vi "histo_alerte.vi"(8 "Error in (no error)":errorcluster, 11 "Connection In":refnum<k7>) -> (0 "Error out":errorcluster, 2 "Table":string[][](table), 3 "Connection Out":refnum<k7>)   [LabVIEW 2019]
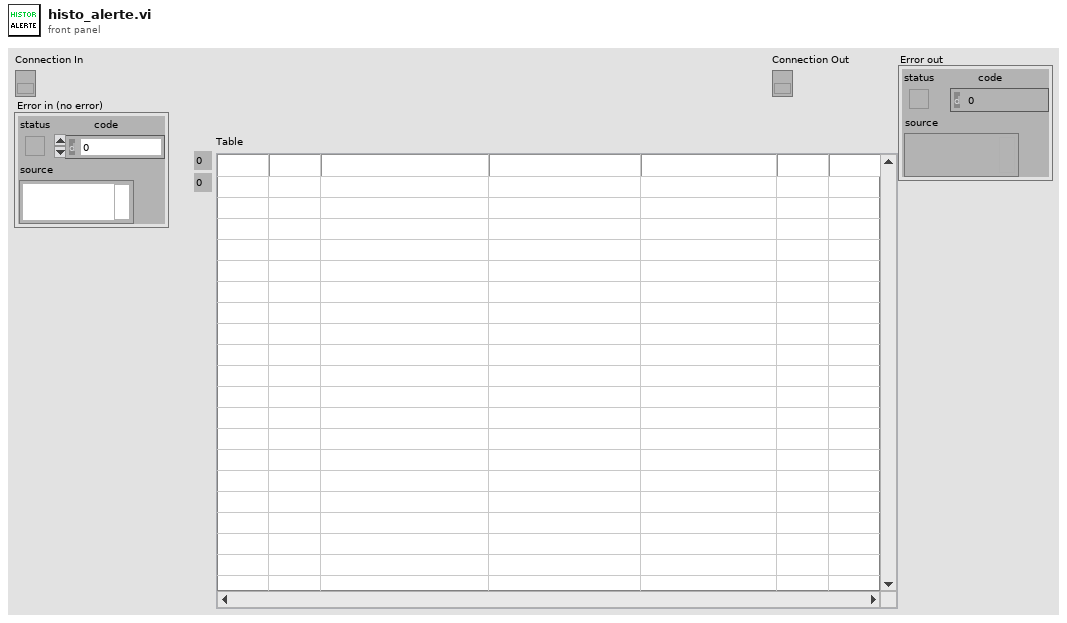
[diagram p1: front panel]
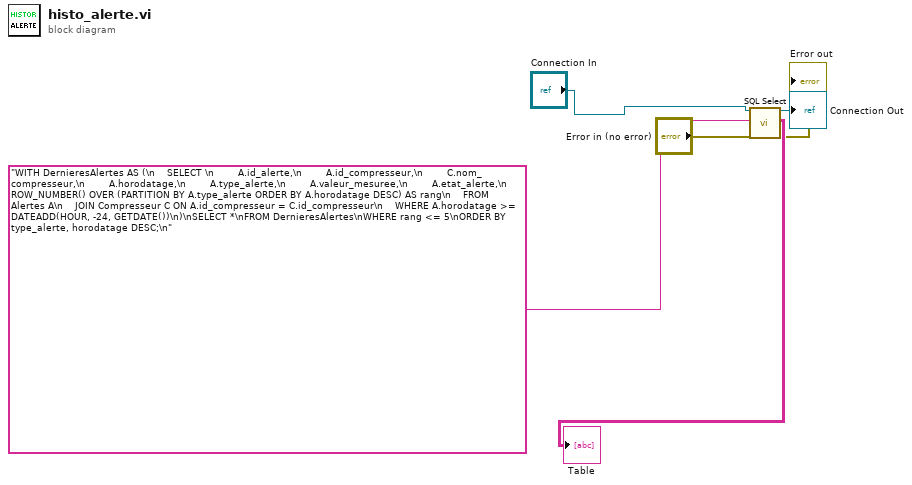
[diagram p0: block diagram]
diagram:
  n1 = call <vilib>:"SQL Select.vi"("Connection In"="Connection In", "SQL Query"="WITH DernieresAlertes AS (\n    SELECT \n        A.id_alerte,\n        A.id_compresseur,\n        C.nom_compresseur,\n        A.horodatage,\n        A.type_alerte,\n        A.valeur_mesuree,\n        A.etat_alerte,\n        ROW_NUMBER() OVER (PARTITION BY A.type_alerte ORDER BY A.horodatage DESC) AS rang\n    FROM Alertes A\n    JOIN Compresseur C ON A.id_compresseur = C.id_compresseur\n    WHERE A.horodatage >= DATEADD(HOUR, -24, GETDATE())\n)\nSELECT *\nFROM DernieresAlertes\nWHERE rang <= 5\nORDER BY type_alerte, horodatage DESC;\n", "Error in (no error)"="Error in (no error)") -> ("Connection Out"=→"Connection Out":refnum<k7>, "Data"=→"Table":string[][], "Error out"=→"Error out":errorcluster)  [unwired: 14 in]
